vi "test_conv3.vi"() -> ()   [LabVIEW 2018]
uses:
  <vilib>/Analysis/1siggen.llb/Ramp Pattern by Samples.vi
  <vilib>/addons/Modulation/Digital/Channel Coding/MT Convolutional Encoder (Rate).vi
  <vilib>/addons/Modulation/Analog/support/mod_Set Error Source.vi
  <vilib>/addons/Modulation/Digital/Support/Common/Validators/mod_Validate Bit Stream.vi
  <vilib>/addons/Modulation/Digital/Channel Coding/Convolutional codes/mod_Convolutional encoder.vi
  <vilib>/addons/Modulation/Digital/Support/Common/Validators/mod_AWGN Validate.vi
  <vilib>/addons/Modulation/Digital/Impairments/subVIs/mod_createSeeds.vi
  <vilib>/addons/Modulation/Digital/Channel Coding/Convolutional codes/subVIs/mod_Generate encoder tap connections.vi
  <vilib>/addons/Modulation/Digital/Channel Coding/Convolutional codes/subVIs/mod_Perform convolutional encoding.vi
  <vilib>/addons/Modulation/Digital/Channel Coding/Block codes/subVIs/mod_Buffer block code info (I8).vi
  <vilib>/addons/Modulation/Digital/Channel Coding/Convolutional codes/subVIs/mod_Generate valid reset (convolutional, I8).vi
  <vilib>/addons/Modulation/Digital/Support/Common/Validators/mod_Validate Samples Per Symbol.vi
  <vilib>/addons/Modulation/Analog/support/Validators/mod_Validate Complex Waveform.vi
  <vilib>/addons/Modulation/Analog/support/Validators/mod_WFErrorHandler.vi
  <vilib>/addons/Modulation/Digital/Support/Common/Validators/mod_Generate Filter Coefficients Validate.vi
  <vilib>/addons/Modulation/Digital/General/subVIs/mod_Generate Filter Coefficients.vi
  <vilib>/addons/Modulation/Digital/General/MT Generate PSK System Parameters(M).vi
  <vilib>/addons/Modulation/Digital/Channel Coding/Convolutional codes/subVIs/mod_Select known generator matrix.vi
  <vilib>/addons/Modulation/Digital/Support/Common/Validators/mod_Validate Convolutional Encoder prms.vi
  <vilib>/addons/Modulation/Digital/General/subVIs/mod_Generate Bits PN Sequence.vi
  <vilib>/Analysis/1siggen.llb/Gaussian White Noise (obs 90).vi
  <vilib>/addons/Modulation/Digital/General/MT Apply Matched Filter (Generic).vi
  <vilib>/addons/Modulation/Digital/General/MT Map PSK Symbols to Bits.vi
  <vilib>/addons/Modulation/Digital/Channel Coding/MT Convolutional Decoder (Viterbi Hard Decision, Rate).vi
  <vilib>/addons/Modulation/niDMT.lvlib
  <vilib>/Analysis/NI_AALBase.lvlib
panel:
  out "CAN":i8[](array[numeric])
  out "dec":i8[](array[numeric])
  out "mes":i8[](array[numeric])
  out "IQ Constellation":T1(graph)
  in  "Traceback Depth (D)":i32=20
  in  "Constraint Length (K)":i32=3
  in  "Rate (k/n)":enum16{"1/2", "1/3", "1/4", "2/3", "3/4"}(ring)
  in  "Trials per Eb/N0 Sample":i32=1
  in  "Start Eb/N0 (dB)":dbl=5.0 format="%0.2f"
  in  "End Eb/N0 (dB)":dbl=10.0 format="%0.2f"
  in  "Eb/N0 Samples":i32=6
  out "Current trial":i32
  out "Current Eb/N0":dbl
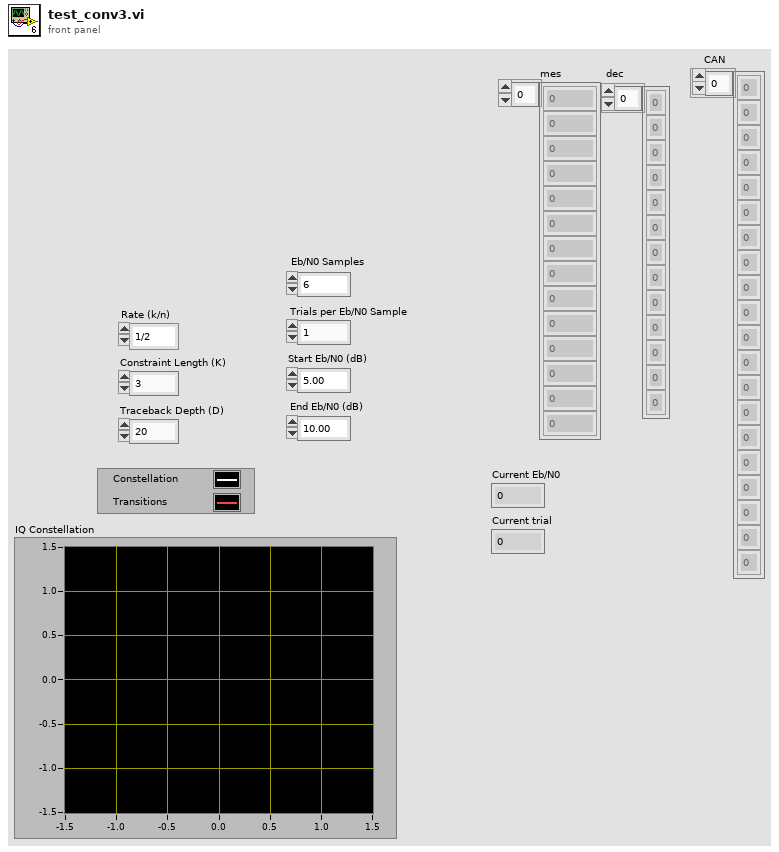
[diagram p1: front panel]
types:
  T1 = cluster{"Decimated Array":dbl[], "Decimated Array":dbl[]}[]
  T2 = enum16{"none", "Raised Cosine", "Root Raised Cos", "Gaussian"}
  T3 = cluster{"samples per symbol (16)":i32, "symbol map":cdb[], "differential PSK":enum16{"disable", "enable"}, "PSK type":u16}
  T4 = typedef "niAMT.lvlib/Complex Data Waveform.ctl" = cluster{"t0":dbl, "dt":dbl, "Y":cdb[]}
  T5 = cluster{"constellation":dbl[], "oversampled data":dbl[]}[]
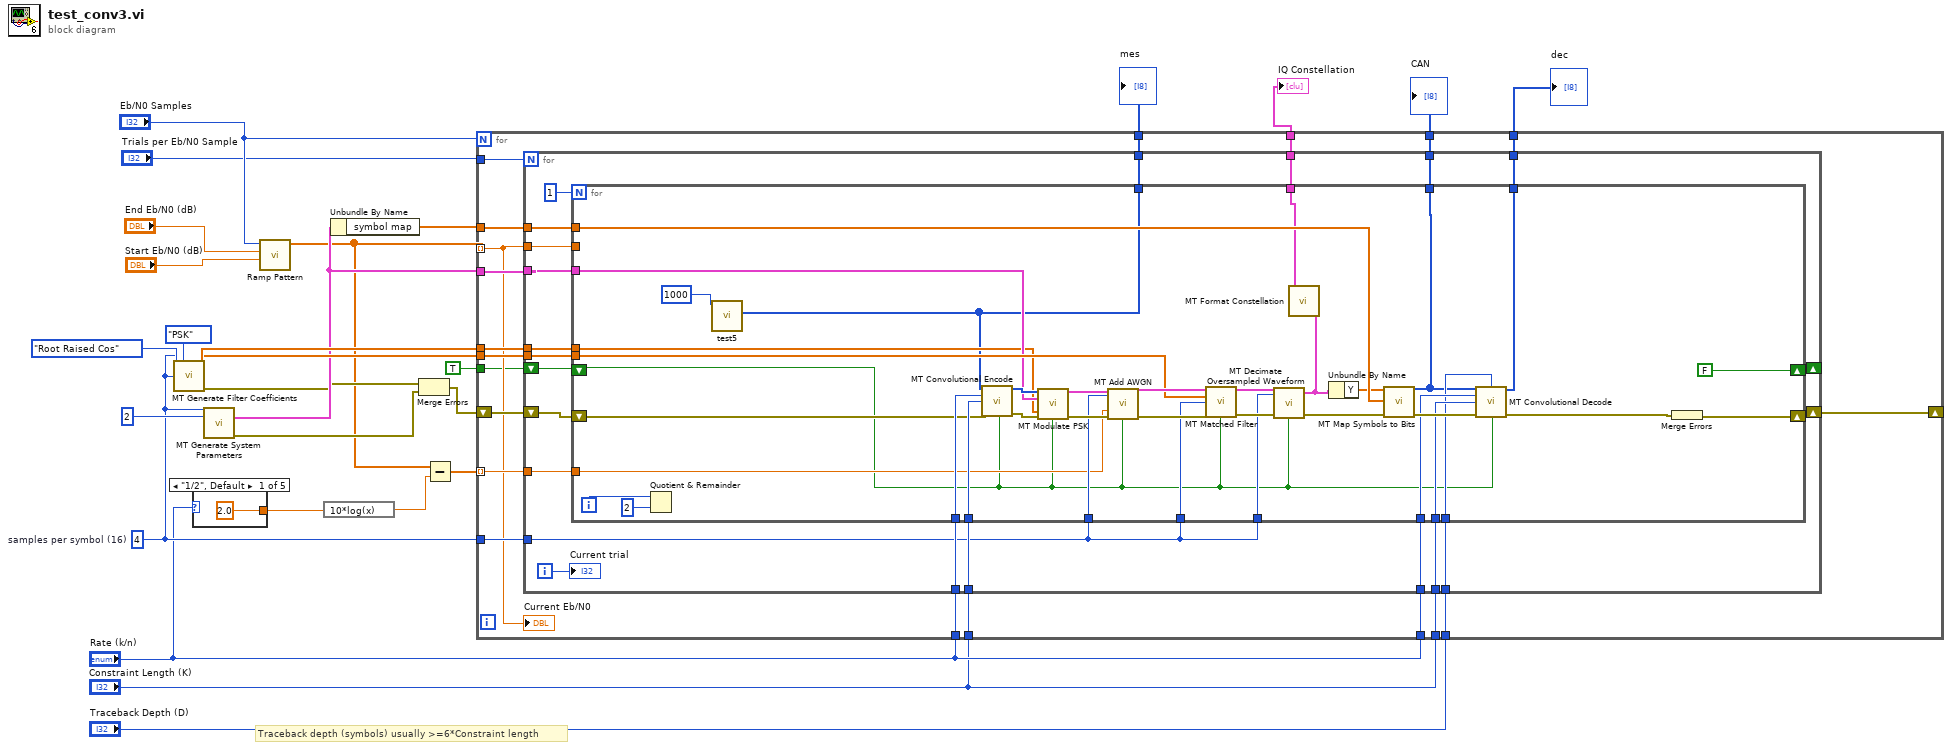
[diagram p0: block diagram]
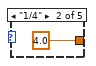
[diagram p2: hidden frame]
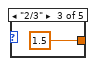
[diagram p3: hidden frame]
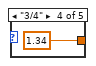
[diagram p4: hidden frame]
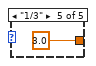
[diagram p5: hidden frame]
diagram:
  w20 = 4  # samples per symbol (16)
  # "Traceback depth (symbols) usually >=6*Constraint length"
  n1 = call <vilib>:"MT Generate Filter Coefficients.vi"("pulse shaping filter (none)"=T2."Root Raised Cos", "modulation type"=enum16{"FSK", "PSK", "QAM", "MSK", "PAM", "ASK"}."PSK", "pulse shaping samples per symbol (16)"=w20, "matched samples per symbol (16)"=w20) -> ("pulse shaping filter coefficients"=w25:dbl[], "matched filter coefficients"=w21:dbl[], "error out"=w15:errorcluster)  [unwired: 9 in]
  n2 = case shown="\"1/2\", Default" "Rate (k/n)" {
    tunnel: [2.0 4.0 1.5 1.34 3.0] -> w10
    frame "1/2", Default {
    }
    frame "1/4" {
    }
    frame "2/3" {
    }
    frame "3/4" {
    }
    frame "1/3" {
    }
  }
  n3 = call-poly <vilib>:"MT Generate System Parameters.vi"("samples per symbol (16)"=w20, "M-PSK (4)"=2) -> ("PSK system parameters"=w19:T3, "error out"=w14:errorcluster)  [unwired: 11 in, 1 out]
  n4 = call-poly <vilib>:"Ramp Pattern.vi"("start"="Start Eb/N0 (dB)", "end"="End Eb/N0 (dB)", "samples"="Eb/N0 Samples") -> ("Ramp Pattern"=w8:dbl[])  [unwired: 7 in, 1 out]
  n5 = expression code="10*log(x)"(w10) -> (w9:dbl)
  n6 = Unbundle By Name(w19) -> ("symbol map"=w18:cdb[])
  n7 = Merge Errors(w15, w14) -> (w13:errorcluster)
  n8 = Subtract(x=w8, y=w9) -> (x-y=w12:dbl[])
  n9 = for {
    N: "Eb/N0 Samples" -> [_]
    tunnel: w25 -> [w52]
    tunnel: "Rate (k/n)" -> [w50]
    tunnel: "Constraint Length (K)" -> [w49]
    tunnel: w8 -> [w38] mode=indexing
    tunnel: w21 -> [w48]
    tunnel: w20 -> [w47]
    tunnel: w18 -> [w46]
    tunnel: "Rate (k/n)" -> [w45]
    tunnel: "Constraint Length (K)" -> [w44]
    tunnel: "Traceback Depth (D)" -> [w43]
    tunnel: "Trials per Eb/N0 Sample" -> [w42]
    tunnel: w19 -> [w51]
    shift-right: [w41] -> _
    shift-left: w13 -> [w40]
    tunnel: w12 -> [w39] mode=indexing
    tunnel: TRUE ("reset? (T)") -> [w37]
    tunnel: [w36] -> w4
    tunnel: [w35] -> w3
    tunnel: [w34] -> w2
    tunnel: [w33] -> w1
    n10 = for {
      N: w42 -> [_]
      tunnel: w52 -> [w74]
      tunnel: w50 -> [w72]
      tunnel: w49 -> [w71]
      tunnel: w38 -> [w70]
      tunnel: w48 -> [w69]
      tunnel: w47 -> [w68]
      tunnel: w46 -> [w67]
      tunnel: w45 -> [w66]
      tunnel: w44 -> [w65]
      tunnel: w43 -> [w64]
      tunnel: w51 -> [w73]
      shift-right: [w61] -> w41
      shift-left: w40 -> [w60]
      tunnel: w39 -> [w59]
      shift-right: [w57] -> _
      shift-left: w37 -> [w58]
      tunnel: [w56] -> w36
      tunnel: [w55] -> w35
      tunnel: [w54] -> w34
      tunnel: [w53] -> w33
      i -> [w62]
      n11 = for {
        N: 1 -> [_]
        tunnel: w74 -> [w87]
        shift-right: [FALSE ("reset? (T)")] -> w57
        shift-left: w58 -> [w79]
        tunnel: w72 -> [w109]
        tunnel: w71 -> [w108]
        tunnel: w70 -> [_]
        tunnel: w69 -> [w105]
        tunnel: w68 -> [w99]
        tunnel: w68 -> [w97]
        tunnel: w68 -> [w98]
        tunnel: w67 -> [w95]
        tunnel: w66 -> [w92]
        tunnel: w65 -> [w91]
        tunnel: w64 -> [w90]
        tunnel: w73 -> [w102]
        shift-right: [w88] -> w61
        shift-left: w60 -> [w82]
        tunnel: w59 -> [w86]
        tunnel: [w78] -> w56
        tunnel: [w77] -> w55
        tunnel: [w76] -> w54
        tunnel: [w75] -> w53
        i -> [w85]
        n12 = Quotient & Remainder(x=w85, y=2) -> ()  [unwired: 2 out]
        n13 = call "test5.vi"("k"=1000) -> ("output bit stream"=w76:i8[])  [unwired: 9 in, 1 out]
        n14 = call-poly <vilib>:"MT Convolutional Encode.vi"("input bit stream"=w76, "rate (k/n)"=w109, "constraint length (K)"=w108, "error in (no error)"=w82, "reset? (T)"=w79) -> ("output bit stream"=w110:i8[], "error out"=w103:errorcluster)  [unwired: 8 in, 1 out]
        n15 = call <vilib>:"MT Modulate PSK.vi"("input bit stream"=w110, "PSK system parameters"=w102, "pulse shaping filter coefficients"=w87, "error in (no error)"=w103, "reset? (T)"=w79) -> ("output complex waveform"=w111:T4, "error out"=w104:errorcluster)  [unwired: 8 in, 1 out]
        n16 = call <vilib>:"MT Add AWGN.vi"("input complex waveform"=w111, "samples per symbol (16)"=w98, "Eb/N0 (10 dB)"=w86, "error in (no error)"=w104, "reset? (T)"=w79) -> ("output complex waveform"=w106:T4, "error out"=w107:errorcluster)  [unwired: 8 in, 1 out]
        n17 = call-poly <vilib>:"MT Matched Filter.vi"("input complex waveform"=w106, "matched filter coefficients"=w105, "samples per symbol (16)"=w97, "error in (no error)"=w107, "reset? (T)"=w79) -> ("output complex waveform"=w101:T4, "error out"=w100:errorcluster)  [unwired: 9 in]
        n18 = call <vilib>:"MT Decimate Oversampled Waveform.vi"("input complex waveform"=w101, "decimation factor"=w99, "error in (no error)"=w100, "reset? (T)"=w79) -> ("output complex waveform"=w83:T4, "error out"=w96:errorcluster)  [unwired: 10 in]
        n19 = call <vilib>:"MT Format Constellation.vi"("waveform"=w83) -> ("constellation graph"=w75:T5)  [unwired: 13 in, 1 out]
        n20 = Unbundle By Name(w83) -> ("Y"=w94:cdb[])
        n21 = call-poly <vilib>:"MT Map Symbols to Bits.vi"("symbols"=w94, "symbol map"=w95, "error in (no error)"=w96) -> ("output bit stream"=w78:i8[], "error out"=w93:errorcluster)  [unwired: 11 in]
        n22 = call-poly <vilib>:"MT Convolutional Decode.vi"("input bit stream"=w78, "traceback depth (D)"=w90, "rate (k/n)"=w92, "constraint length (K)"=w91, "error in (no error)"=w93, "reset? (T)"=w79) -> ("output bit stream"=w77:i8[], "error out"=w80:errorcluster)  [unwired: 7 in, 1 out]
        n23 = Merge Errors(w80) -> (w88:errorcluster)
      }
      "Current trial" <- w62
    }
    "Current Eb/N0" <- w38
  }
  "CAN" <- w4
  "dec" <- w3
  "mes" <- w2
  "IQ Constellation" <- w1
